vi "FVB32at.vi"() -> ()   [LabVIEW 2019]
panel:
  out "Waveform Graph":i32[](graph)
  out "Detector Y Pixels":i32
  in  "Shut Down":bool
  in  "Start Acquisition":bool
  out "Return  from Get Acquired Data":u32
  out "Detector X Pixels":i32
  out "Return from GetStatus":u32
  out "Return from Start Acquisition":u32
  out "Return from CheckTimings":u32
  out "Calculated Exposure Value":sgl format="%.2f"
  in  "Exposure Time (secs)":sgl=0.05 format="%.2f"
  out "Return from Initialize":u32
  in  "Trigger":u32(ring) items=["Internal", "External"]
  # "Acquisition Mode: Single Scan\nReadout Mode: Full Vertical Binning\nCools to desired temperature, acquires data and then brings the temperature up to 0 in a controlled way."
  # "Status"
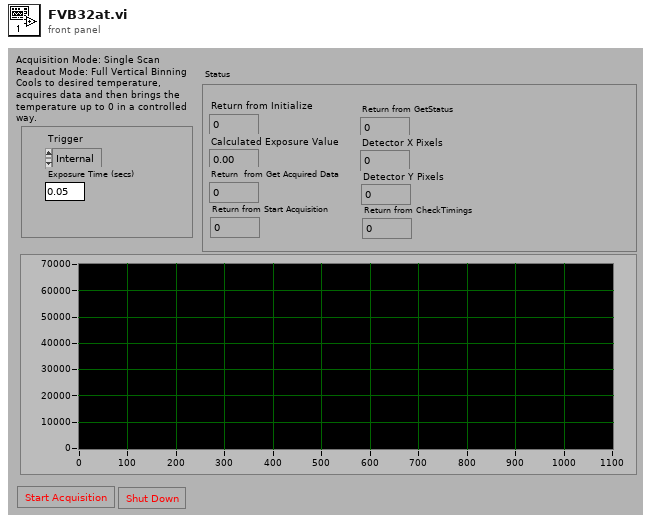
[diagram p1: front panel]
types:
  T1 = typedef "Error Code Enum typedef.ctl" = enum32{"N/A (0)", "DRV_ERROR_CODES", "DRV_SUCCESS", "DRV_VXDNOTINSTALLED", "DRV_ERROR_SCAN", "DRV_ERROR_CHECK_SUM", "DRV_ERROR_FILELOAD", "DRV_UNKNOWN_FUNC", "DRV_ERROR_VXD_INIT", "DRV_ERROR_ADDRESS", "DRV_ERROR_PAGELOCK", "DRV_ERROR_PAGEUNLOCK", "DRV_ERROR_BOARDTEST", "DRV_ERROR_ACK", "DRV_ERROR_UP_FIFO", "DRV_ERROR_PATTERN", "N/A (16)", "DRV_ACQUISITION_ERRORS", "DRV_ACQ_BUFFER", "DRV_ACQ_DOWNFIFO_FULL", "DRV_PROC_UNKONWN_INSTRUCTION", "DRV_ILLEGAL_OP_CODE", "DRV_KINETIC_TIME_NOT_MET", "DRV_ACCUM_TIME_NOT_MET", "DRV_NO_NEW_DATA", "N/A (25)", "DRV_SPOOLERROR", "N/A (27)", "N/A (28)", "N/A (29)", "N/A (30)", "N/A (31)", "N/A (32)", "DRV_TEMPERATURE_CODES", "DRV_TEMPERATURE_OFF", "DRV_TEMPERATURE_NOT_STABILIZED", "DRV_TEMPERATURE_STABILIZED", "DRV_TEMPERATURE_NOT_REACHED", "DRV_TEMPERATURE_OUT_RANGE", "DRV_TEMPERATURE_NOT_SUPPORTED", "DRV_TEMPERATURE_DRIFT", "N/A (41)", "N/A (42)", "N/A (43)", "N/A (44)", "N/A (45)", "N/A (46)", "N/A (47)", "N/A (48)", "DRV_GENERAL_ERRORS", "DRV_INVALID_AUX", "DRV_COF_NOTLOADED", "DRV_FPGAPROG", "DRV_FLEXERROR", "DRV_GPIBERROR", "N/A (55)", "N/A (56)", "N/A (57)", "N/A (58)", "N/A (59)", "N/A (60)", "N/A (61)", "N/A (62)", "N/A (63)", "DRV_DATATYPE", "DRV_DRIVER_ERRORS", "DRV_P1INVALID", "DRV_P2INVALID", "DRV_P3INVALID", "DRV_P4INVALID", "DRV_INIERROR", "DRV_COFERROR", "DRV_ACQUIRING", "DRV_IDLE", "DRV_TEMPCYCLE", "DRV_NOT_INITIALIZED", "DRV_P5INVALID", "DRV_P6INVALID", "DRV_INVALID_MODE", "DRV_INVALID_FILTER", "DRV_I2CERRORS", "DRV_I2CDEVNOTFOUND", "DRV_I2CTIMEOUT", "DRV_P7INVALID", "N/A (84)", "N/A (85)", "N/A (86)", "N/A (87)", "N/A (88)", "N/A (89)", "DRV_IOCERROR", "DRV_VRMVERSIONERROR"}
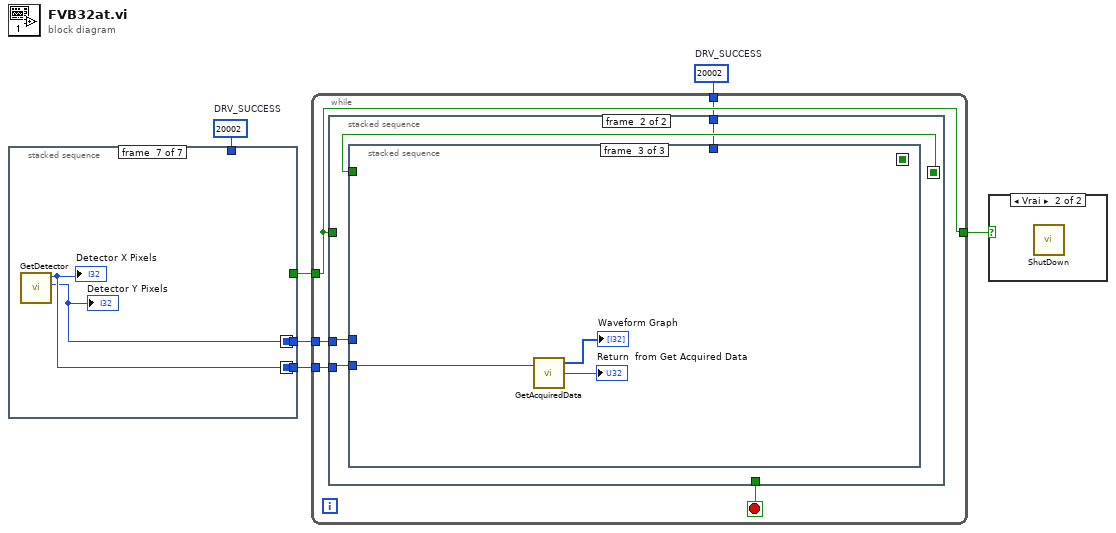
[diagram p0: block diagram]
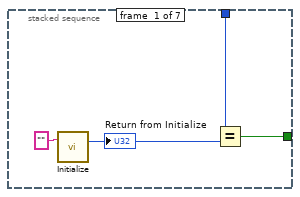
[diagram p3: hidden frame]
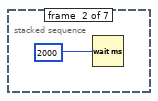
[diagram p4: hidden frame]
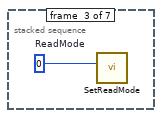
[diagram p5: hidden frame]
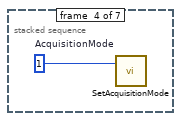
[diagram p6: hidden frame]
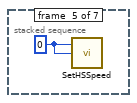
[diagram p7: hidden frame]
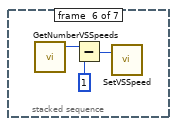
[diagram p8: hidden frame]
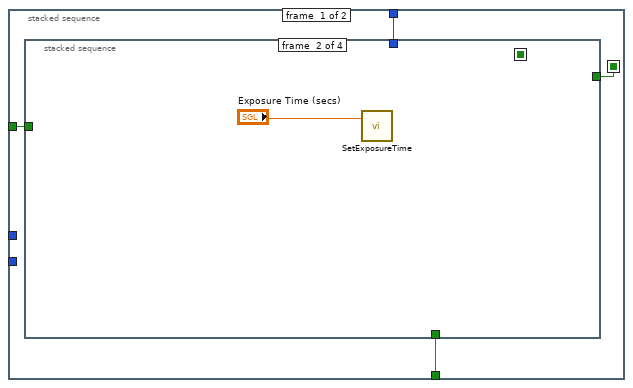
[diagram p9: hidden frame]
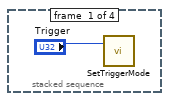
[diagram p10: hidden frame]
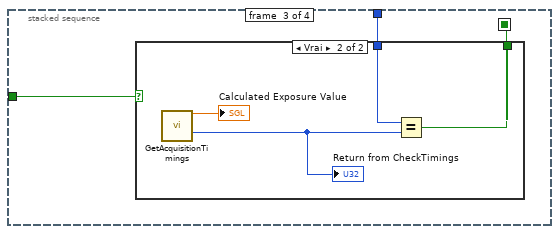
[diagram p11: hidden frame]
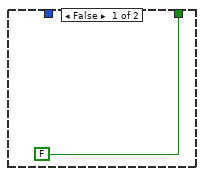
[diagram p12: hidden frame]
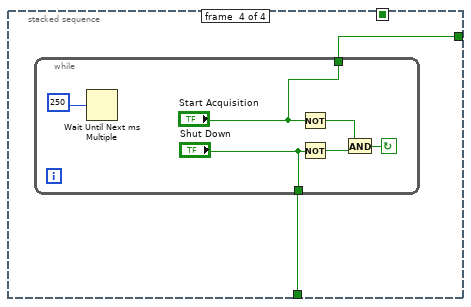
[diagram p13: hidden frame]
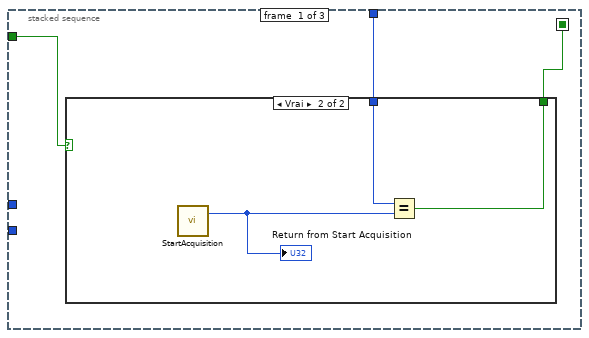
[diagram p14: hidden frame]
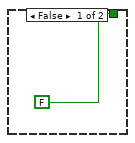
[diagram p15: hidden frame]
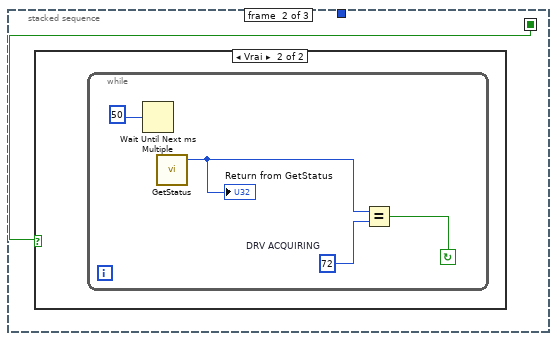
[diagram p16: hidden frame]
diagram:
  w1 = 20002  # DRV_SUCCESS
  w5 = 20002  # DRV_SUCCESS
  n1 = stacked-sequence {
    seq-local: [_ _ _ _ _ _ w18] -> [_ _ _ _ _ _ _]
    seq-local: [_ _ _ _ _ _ w19] -> [_ _ _ _ _ _ _]
    tunnel: w5 -> [w8 _ _ _ _ _ _]
    tunnel: [w7 _ _ _ _ _ _] -> w4
    tunnel: [_ _ _ _ _ _ w18] -> w3
    tunnel: [_ _ _ _ _ _ w19] -> w2
    frame #0 {
      n2 = call <userlib>:"Initialize.vi"("directory (\"\")"="" ("directory (\"\")")) -> ("DLL error code"=w10:u32)  [unwired: 1 in, 1 out]
      "Return from Initialize" <- w10
      n3 = Equal?(x=w8, y=w10) -> (x = y?=w7:bool)
    }
    frame #1 {
      n4 = Wait (ms)(milliseconds to wait=u32 2000) -> ()  [unwired: 1 out]
    }
    frame #2 {
      w12 = u16 0  # ReadMode
      n5 = call <userlib>:"SetReadMode.vi"("mode"=w12) -> ()  [unwired: 1 in, 2 out]
    }
    frame #3 {
      w13 = u16 1  # AcquisitionMode
      n6 = call <userlib>:"SetAcquisitionMode.vi"("mode"=w13) -> ()  [unwired: 1 in, 2 out]
    }
    frame #4 {
      w14 = 0
      n7 = call <userlib>:"SetHSSpeed.vi"("index"=w14, "type"=w14) -> ()  [unwired: 2 in, 2 out]
    }
    frame #5 {
      n8 = call <userlib>:"GetNumberVSSpeeds.vi"() -> ("number"=w17:i32)  [unwired: 3 in, 2 out]
      n9 = Subtract(x=w17, y=1) -> (x-y=w15:i32)
      n10 = call <userlib>:"SetVSSpeed.vi"("index"=w15) -> ()  [unwired: 1 in, 2 out]
    }
    frame #6 {
      n11 = call <userlib>:"GetDetector.vi"() -> ("ypixels"=w18:i32, "xpixels"=w19:i32)  [unwired: 4 in, 2 out]
      "Detector Y Pixels" <- w18
      "Detector X Pixels" <- w19
    }
  }
  n12 = while {
    tunnel: [w21] -> w6
    tunnel: w4 -> [w21]
    tunnel: w3 -> [w24]
    tunnel: w2 -> [w23]
    tunnel: w1 -> [w20]
    stop <- w22 stop-if-true
    n13 = stacked-sequence {
      seq-local: [w28 _] -> [_ w50]
      tunnel: w24 -> [_ w49]
      tunnel: w23 -> [_ w48]
      tunnel: [w27 _] -> w22
      tunnel: w21 -> [w26 _]
      tunnel: w20 -> [w25 w47]
      frame #0 {
        n14 = stacked-sequence {
          seq-local: [_ _ w32 _] -> [_ _ _ _]
          tunnel: w25 -> [_ _ w33 _]
          tunnel: [_ _ _ w40] -> w28
          tunnel: [_ _ _ w39] -> w27
          tunnel: w26 -> [_ _ w31 _]
          frame #0 {
            n15 = call <userlib>:"SetTriggerMode.vi"("mode"="Trigger") -> ()  [unwired: 1 in, 2 out]
          }
          frame #1 {
            n16 = call <userlib>:"SetExposureTime.vi"("time"="Exposure Time (secs)") -> ()  [unwired: 1 in, 2 out]
          }
          frame #2 {
            n17 = case shown="Vrai" w31 {
              tunnel: w33 -> [_ w36]
              tunnel: [FALSE w38] -> w32
              frame False {
              }
              frame True {
                n18 = call <userlib>:"GetAcquisitionTimings.vi"() -> ("exposure"=→"Calculated Exposure Value":sgl, "DLL error code"=w35:u32)  [unwired: 11 in, 3 out]
                "Return from CheckTimings" <- w35
                n19 = Equal?(x=w36, y=w35) -> (x = y?=w38:bool)
              }
            }
          }
          frame #3 {
            n20 = while {
              tunnel: ["Shut Down"] -> w39
              tunnel: ["Start Acquisition"] -> w40
              stop <- w43 continue-if-true
              n21 = Wait Until Next ms Multiple(millisecond multiple=u32 250) -> ()  [unwired: 1 out]
              n22 = Not(x="Start Acquisition") -> (.not. x?=w44:bool)
              n23 = Not(x="Shut Down") -> (.not. x?=w45:bool)
              n24 = And(x=w44, y=w45) -> (x .and. y?=w43:bool)
            }
          }
        }
      }
      frame #1 {
        n25 = stacked-sequence {
          seq-local: [w52 _ _] -> [_ w58 _]
          tunnel: w47 -> [w53 _ _]
          tunnel: w50 -> [w51 _ _]
          tunnel: w49 -> [_ _ _]
          tunnel: w48 -> [_ _ w64]
          frame #0 {
            n26 = case shown="Vrai" w51 {
              tunnel: [FALSE w57] -> w52
              tunnel: w53 -> [_ w56]
              frame False {
              }
              frame True {
                n27 = call <userlib>:"StartAcquisition.vi"() -> ("DLL error code"=w55:u32)  [unwired: 2 in, 1 out]
                "Return from Start Acquisition" <- w55
                n28 = Equal?(x=w56, y=w55) -> (x = y?=w57:bool)
              }
            }
          }
          frame #1 {
            n29 = case shown="Vrai" w58 {
              frame False {
              }
              frame True {
                n30 = while {
                  stop <- w61 continue-if-true
                  w60 = u16 72  # DRV ACQUIRING
                  n31 = Wait Until Next ms Multiple(millisecond multiple=u32 50) -> ()  [unwired: 1 out]
                  n32 = call <userlib>:"GetStatus.vi"() -> ("status"=w59:T1)  [unwired: 3 in, 2 out]
                  "Return from GetStatus" <- w59
                  n33 = Equal?(x=w59, y=w60) -> (x = y?=w61:bool)
                }
              }
            }
          }
          frame #2 {
            n34 = call <userlib>:"GetAcquiredData.vi"("size"=w64) -> ("DLL error code"=→"Return  from Get Acquired Data":u32, "array"=→"Waveform Graph":i32[])  [unwired: 2 in, 1 out]
          }
        }
      }
    }
  }
  n35 = case shown="Vrai" w6 {
    frame False {
    }
    frame True {
      n36 = call <userlib>:"ShutDown.vi"() -> ()  [unwired: 2 in, 2 out]
    }
  }
